vi "全局断电保存变量.vi"() -> ()   [LabVIEW 2016, in "main.lvlib"]
uses:
  main.lvlib
  control/checkbox.ctl
panel:
  in  "手动湖面水深设置值":sgl=9.0
  in  "水深获取方式":bool caption="自动/手动获取湖面水深"
  in  "仪器类型":enum16{"EXO2", "BBE+NAQDO"}(ring)
  in  "DO启用":T1 caption="启用"
  in  "BBE启用":T1 caption="启用"
  in  "BBE串口":refnum<visa-resource-name>
  in  "计数器启用":T1 caption="启用"
  in  "声纳启用":T1 caption="启用"
  in  "EXO2启用":T1 caption="启用"
  in  "计数器串口":refnum<visa-resource-name>
  in  "声纳串口":refnum<visa-resource-name>
  in  "EXO2baud rate (9600)":u32=9600 caption="波特率"
  in  "EXO2串口":refnum<visa-resource-name>
  in  "测试间隔":u16=4
  in  "周期运行":bool
  in  "软限位最大值":dbl=25.0 format="%#_6f m"
  in  "软限位最小值":dbl=1.0 format="%#_6f m"
  in  "单层监测时间":u16=60 format="%.0f s"
  in  "剖面单层深度设置":dbl=1.0 format="%#_6f m"
  in  "剖面底层最小深度设定":dbl=2.0 format="%#_6f m"
  in  "剖面第一层位置设定":dbl=2.0 format="%#_6f m"
  in  "剖面待机位置设定":dbl=2.0 format="%#_6f m"
  in  "剖面位置校正值":dbl format="%#_6f m"
  in  "编码器工程变换系数_工程值":dbl=0.251327 format="%#_6f m"
  in  "编码器工程变换系数_计数值":dbl=360.0 format="%#_6f ps"
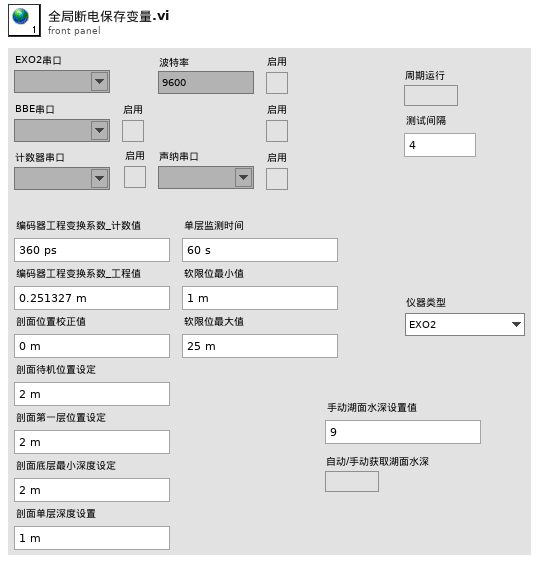
[diagram p1: front panel]
types:
  T1 = typedef "checkbox.ctl" = bool
diagram:
